vi "Publish Sample.vi"(8 "error in (no error)":errorcluster, 10 "Sample":refnum<class "Sample.lvclass">, 11 "Syringe Line in":refnum<class "Syringe Line.lvclass">) -> (0 "error out":errorcluster, 3 "Syringe Line out":refnum<class "Syringe Line.lvclass">)   [LabVIEW 2015, in "cRIO-Carbondioxide.lvlib" / "CO2-Actor.lvlib" / "Syringe Line.lvclass"]
uses:
  Syringe Line.lvclass
  subs/Sample/Sample.lvclass
  Syringe Line.lvclass/Syringe Line.ctl
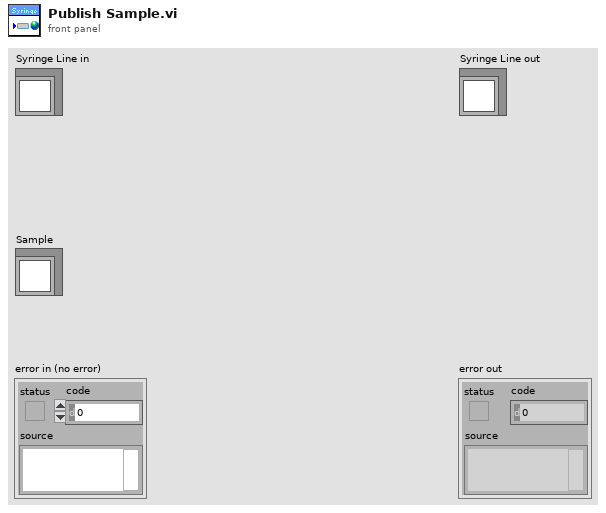
[diagram p1: front panel]
types:
  T1 = typedef "Sample Container.ctl" = cluster{"Sample In":refnum<k21>, "Sample Name":refnum<k21>, "Ti Cathode":refnum<k21>, "SampleQ":refnum<queue>}
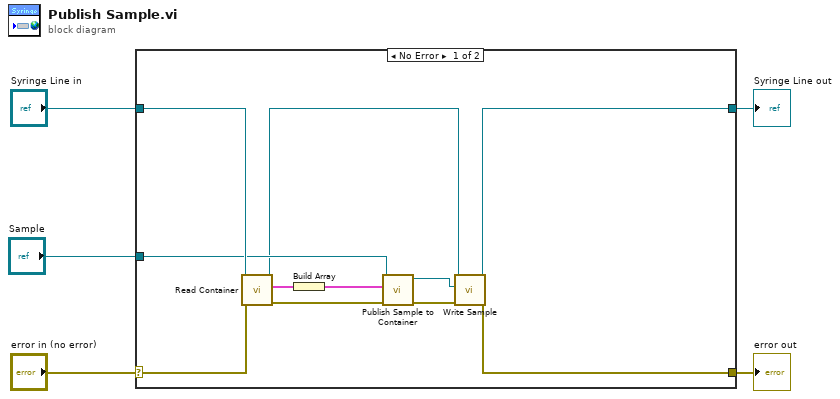
[diagram p0: block diagram]
diagram:
  n1 = case shown="No Error" "error in (no error)" {
    selector: "error in (no error)" -> [w16 w18]
    tunnel: [w7 w18] -> w4
    tunnel: [w9 w17] -> w2
    tunnel: "Syringe Line in" -> [w15 w17]
    tunnel: "Sample" -> [w12 _]
    frame No Error {
      n2 = call "Read Container.vi"("error in (no error)"=w16, "Syringe Line in"=w15) -> ("error out"=w8:errorcluster, "Container"=w14:T1, "Syringe Line out"=w10:refnum<class "Syringe Line.lvclass">)  [unwired: 6 in, 1 out]
      n3 = Build Array(w14) -> (w13:T1[])
      n4 = call "Publish Sample to Container.vi"("error in (no error)"=w8, "Containers"=w13, "Sample in"=w12) -> ("error out"=w11:errorcluster, "Sample out"=w6:refnum<class "Sample.lvclass">)  [unwired: 7 in]
      n5 = call "Write Sample.vi"("error in (no error)"=w11, "Sample"=w6, "Syringe Line in"=w10) -> ("error out"=w7:errorcluster, "Syringe Line out"=w9:refnum<class "Syringe Line.lvclass">)  [unwired: 7 in]
    }
    frame Error {
    }
  }
  "error out" <- w4
  "Syringe Line out" <- w2
